vi "Shutdown CSV.vi"(8 "error in (no error)":errorcluster, 11 "Hardware Resources in":T1={"State"=enum."Idle S3DK", "Settings"="", "Online"=FALSE, "S3DK"={"Signals"={"Phasor"=[], "Analog"=[], "Digital"=[]}}, "CSV"={"Index"=0, "Parcel Length"=0, "EOF?"=FALSE, "Config"={"Mode"=enum."Full timestamp", "delimiter (\\t)"="\t", "Path"=path "", "Rectangular?"=FALSE}}}) -> (0 "error out":errorcluster)   [LabVIEW 2017, in "Acquisition.lvlib"]
doc: "Stops the acquisition."
uses:
  Acquisition.lvlib
  Acquisition Settings.ctl
  Acquisition State.ctl
  support/libs/CSV Reader/Mode CSV reader.ctl
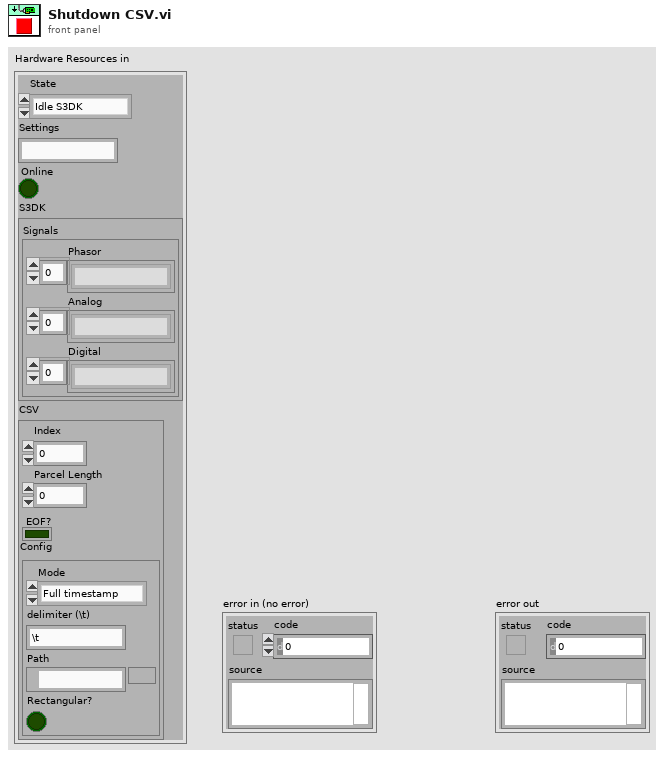
[diagram p1: front panel]
types:
  T1 = typedef "Acquisition.lvlib/Acquisition Settings.ctl" = cluster{"State":T2, "Settings":string, "Online":bool, "S3DK":cluster{"Signals":cluster{"Phasor":string[], "Analog":string[], "Digital":string[]}}, "CSV":cluster{"Index":i32, "Parcel Length":i32, "EOF?":bool, "Config":cluster{"Mode":T3, "delimiter (\\t)":string, "Path":path, "Rectangular?":bool}}}
  T2 = typedef "Acquisition.lvlib/Acquisition State.ctl" = enum16{"Idle", "Idle S3DK", "Acquiring S3DK", "Idle CSV", "Acquiring CSV"}
  T3 = typedef "Mode CSV reader.ctl" = enum16{"Full timestamp", "Relative Time", "Seconds Time", "Nanoseconds Time"}
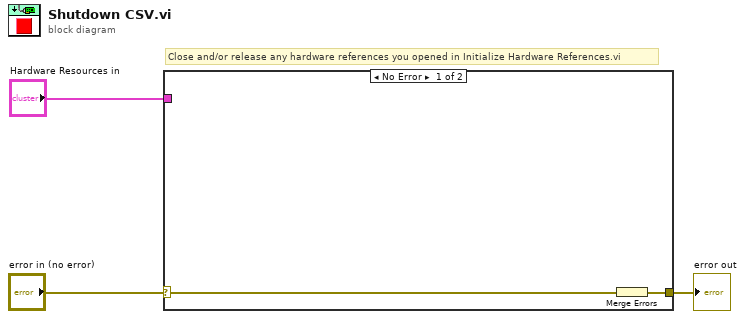
[diagram p0: block diagram]
diagram:
  # "Close and/or release any hardware references you opened in Initialize Hardware References.vi"
  n1 = case shown="No Error" "error in (no error)" {
    selector: "error in (no error)" -> [w4 w6]
    tunnel: [w5 w6] -> w2
    tunnel: "Hardware Resources in" -> [_ _]
    frame No Error {
      n2 = Merge Errors(w4) -> (w5:errorcluster)
    }
    frame Error {
    }
  }
  "error out" <- w2
